vi "Get_Controls.vi"(1 "VI Reference":refnum<vi>) -> (0 "Controls":refnum<vi>[](array[refnum]))   [LabVIEW 2011]
doc: "This VI takes a VI Refernece and returns an array containing all controls on that VI, including those contained within Tab Controls."
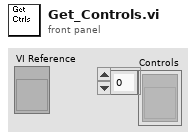
[diagram p1: front panel]
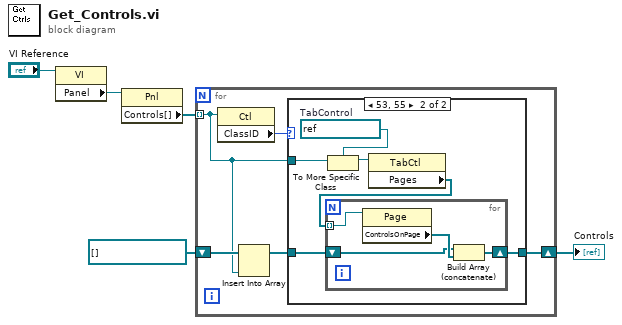
[diagram p0: block diagram]
diagram:
  n1 = property class="VI"(reference="VI Reference") -> ("Panel"=w5:refnum<vi>)  [unwired: 1 in, 2 out]
  n2 = property class="Pnl"(reference=w5) -> ("Controls[]"=w4:refnum<vi>[])  [unwired: 1 in, 2 out]
  n3 = for {
    tunnel: w4 -> [w6] mode=indexing
    shift-right: [w9] -> w1
    shift-left: refnum<vi>[] [] -> [w8]
    n4 = property class="Ctl"(reference=w6) -> ("ClassID"=w10:u32)  [unwired: 1 in, 2 out]
    n5 = Insert Into Array(array=w8, new element=w6) -> (w7:refnum<vi>[])  [unwired: 1 in]
    n6 = case shown="53, 55" w10 {
      tunnel: w6 -> [_ w17]
      tunnel: w7 -> [w11 w13]
      tunnel: [w11 w12] -> w9
      frame Default {
      }
      frame 53, 55 {
        w16 = refnum<vi> refnum  # TabControl
        n7 = To More Specific Class(target class=w16, reference=w17) -> (specific class reference=w15:refnum<vi>)  [unwired: 1 in, 1 out]
        n8 = property class="TabCtl"(reference=w15) -> ("Pages"=w14:refnum<vi>[])  [unwired: 1 in, 2 out]
        n9 = for {
          tunnel: w14 -> [w21] mode=indexing
          shift-right: [w19] -> w12
          shift-left: w13 -> [w18]
          n10 = property class="Page"(reference=w21) -> ("ControlsOnPage"=w20:refnum<vi>[])  [unwired: 1 in, 2 out]
          n11 = Build Array (concatenate)(w18, w20) -> (w19:refnum<vi>[])
        }
      }
    }
  }
  "Controls" <- w1
